vi "Configure Logic Trigger Inputs.vi"(0 "VISA Resource Name":refnum<visa-resource-name>, 1 "Threshold 1 (4.0 V)":dbl=4.0 format="%.2p", 2 "High Logic Level 1 (True)":bool=TRUE, 5 "Input 1 (\"CH1\")":string(combo)="CH1", 9 "Input 2 (\"CH2\")":string(combo)="CH2", 11 "error in (no error)":errorcluster {"code" format="%.0x"}, 12 "Threshold 2 (4.0 V)":dbl=4.0 format="%.2p", 13 "High Logic Level 2 (True)":bool=TRUE) -> (4 "VISA Resource Name Out":refnum<visa-resource-name>, 15 "error out":errorcluster {"code" format="%.0x"})   [LabVIEW 2010, in "Tektronix TDS 3000 Series.lvlib"]
doc: "This VI configures the scope for logic triggering. You configure the controls for the state and pattern triggering.\n\nNotes:\n(1) After configuring the input channels for the logic trigger, call either Configure State Trigger or Configure Pattern Trigger according to the trigger type selected for Trigger Type control in Configure Trigger VI."
uses:
  <instrlib>/Tektronix TDS 3000 Series/Tektronix TDS 3000 Series.lvlib
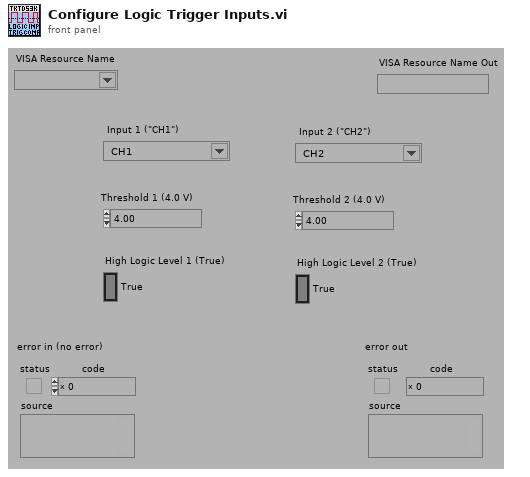
[diagram p1: front panel]
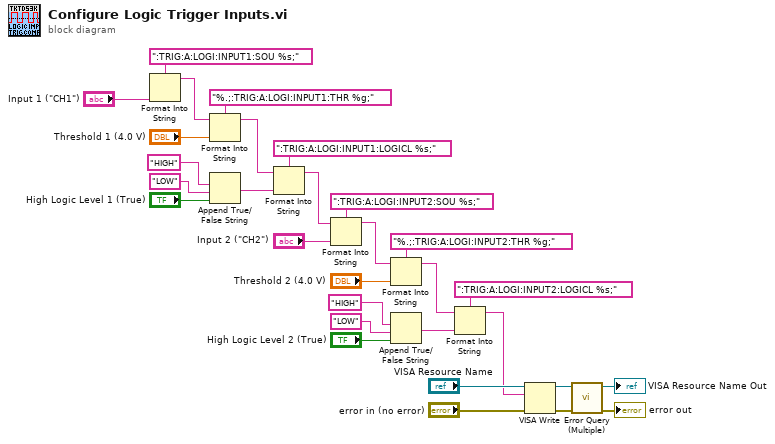
[diagram p0: block diagram]
diagram:
  n1 = Format Into String(format string=":TRIG:A:LOGI:INPUT1:SOU %s;", "Input 1 (\"CH1\")") -> (resulting string=w21:string)  [unwired: 2 in, 1 out]
  n2 = Format Into String(format string="%.;:TRIG:A:LOGI:INPUT1:THR %g;", initial string=w21, "Threshold 1 (4.0 V)") -> (resulting string=w19:string)  [unwired: 1 in, 1 out]
  n3 = Append True/False String(1:"High Logic Level 1 (True)", 2:"LOW" ("false string"), 3:"HIGH" ("true string")) -> (0:w18:string)  [unwired: 1 in]
  n4 = Format Into String(format string=":TRIG:A:LOGI:INPUT1:LOGICL %s;", initial string=w19, w18) -> (resulting string=w6:string)  [unwired: 1 in, 1 out]
  n5 = Format Into String(format string=":TRIG:A:LOGI:INPUT2:SOU %s;", initial string=w6, "Input 2 (\"CH2\")") -> (resulting string=w14:string)  [unwired: 1 in, 1 out]
  n6 = Format Into String(format string="%.;:TRIG:A:LOGI:INPUT2:THR %g;", initial string=w14, "Threshold 2 (4.0 V)") -> (resulting string=w16:string)  [unwired: 1 in, 1 out]
  n7 = Append True/False String(1:"High Logic Level 2 (True)", 2:"LOW" ("false string"), 3:"HIGH" ("true string")) -> (0:w17:string)  [unwired: 1 in]
  n8 = Format Into String(format string=":TRIG:A:LOGI:INPUT2:LOGICL %s;", initial string=w16, w17) -> (resulting string=w5:string)  [unwired: 1 in, 1 out]
  n9 = VISA Write(VISA resource name="VISA Resource Name", write buffer=w5, error in (no error)="error in (no error)") -> (VISA resource name out=w4:refnum<visa-resource-name>, error out=w3:errorcluster)  [unwired: 1 out]
  n10 = call <instrlib>:"Error Query (Multiple).vi"("error in (no error)"=w3, "VISA Resource Name"=w4) -> ("error out"=→"error out":errorcluster, "VISA Resource Name Out"=→"VISA Resource Name Out":refnum<visa-resource-name>)  [unwired: 6 in, 2 out]
